vi "B_humid_air_T_2024.vi"(6 "Bdw source air-water interaction virial":i32(listbox)=3, 8 "Bw source ref water":i32(listbox)=2, 9 "Bd source ref dry air":i32(listbox)=1, 10 "xw molar fraction water vapor":dbl=0.8014618300221631 format="%.6g", 11 "Temperature (K)":dbl=373.15 format="%.4g") -> (0 "Bhumid air (xw,T) [m^3/mol]":dbl=-0.0002943870785351169, 1 "Bdw(T) [m^3/mol]":dbl=-1.3917800082878983e-05, 2 "Bw(T) [m^3/mol]":dbl=-0.00045162277028342796, 3 "Bd(T) [m^3/mol]":dbl=3.5008568678367798e-06, 4 "u(Bdw) [cm^3/mol]":dbl=1.0000812523517617 format="%_3g")   [LabVIEW 2016]
uses:
  2022/SOS_Global_2022.vi
  <vilib>/gmath/NI_Gmath.lvlib
  <vilib>/Analysis/NI_AALPro.lvlib
panel:
  out "Bdw(T) [cm^3/mol]":dbl=-13.917800082878983 format="%_6g"
  in  "interpolation method":i32(ring)=2 items=["nearest", "linear", "spline", "cubic Hermite", "Lagrange"]
  in  "interpolation method":i32(ring)=2 items=["nearest", "linear", "spline", "cubic Hermite", "Lagrange"]
  out "Bhumid air (xw,T) [cm^3/mol]":dbl=-294.38707853511687 format="%_6g"
  out "Bw(T) [cm^3/mol]":dbl=-451.62277028342794 format="%_6g"
  out "Bd(T) [cm^3/mol]":dbl=3.50085686783678
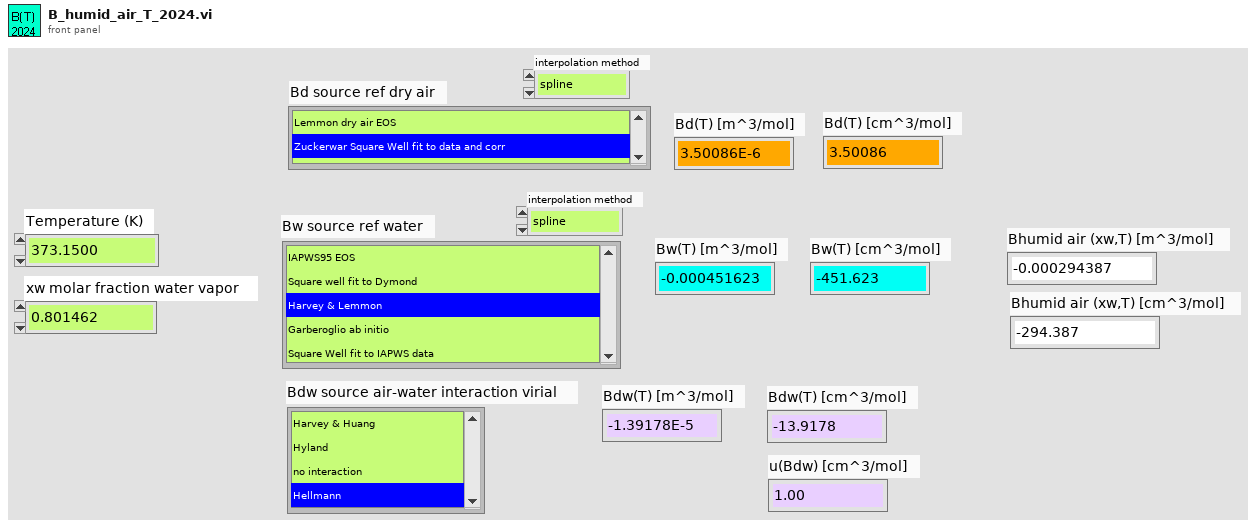
[diagram p1: front panel]
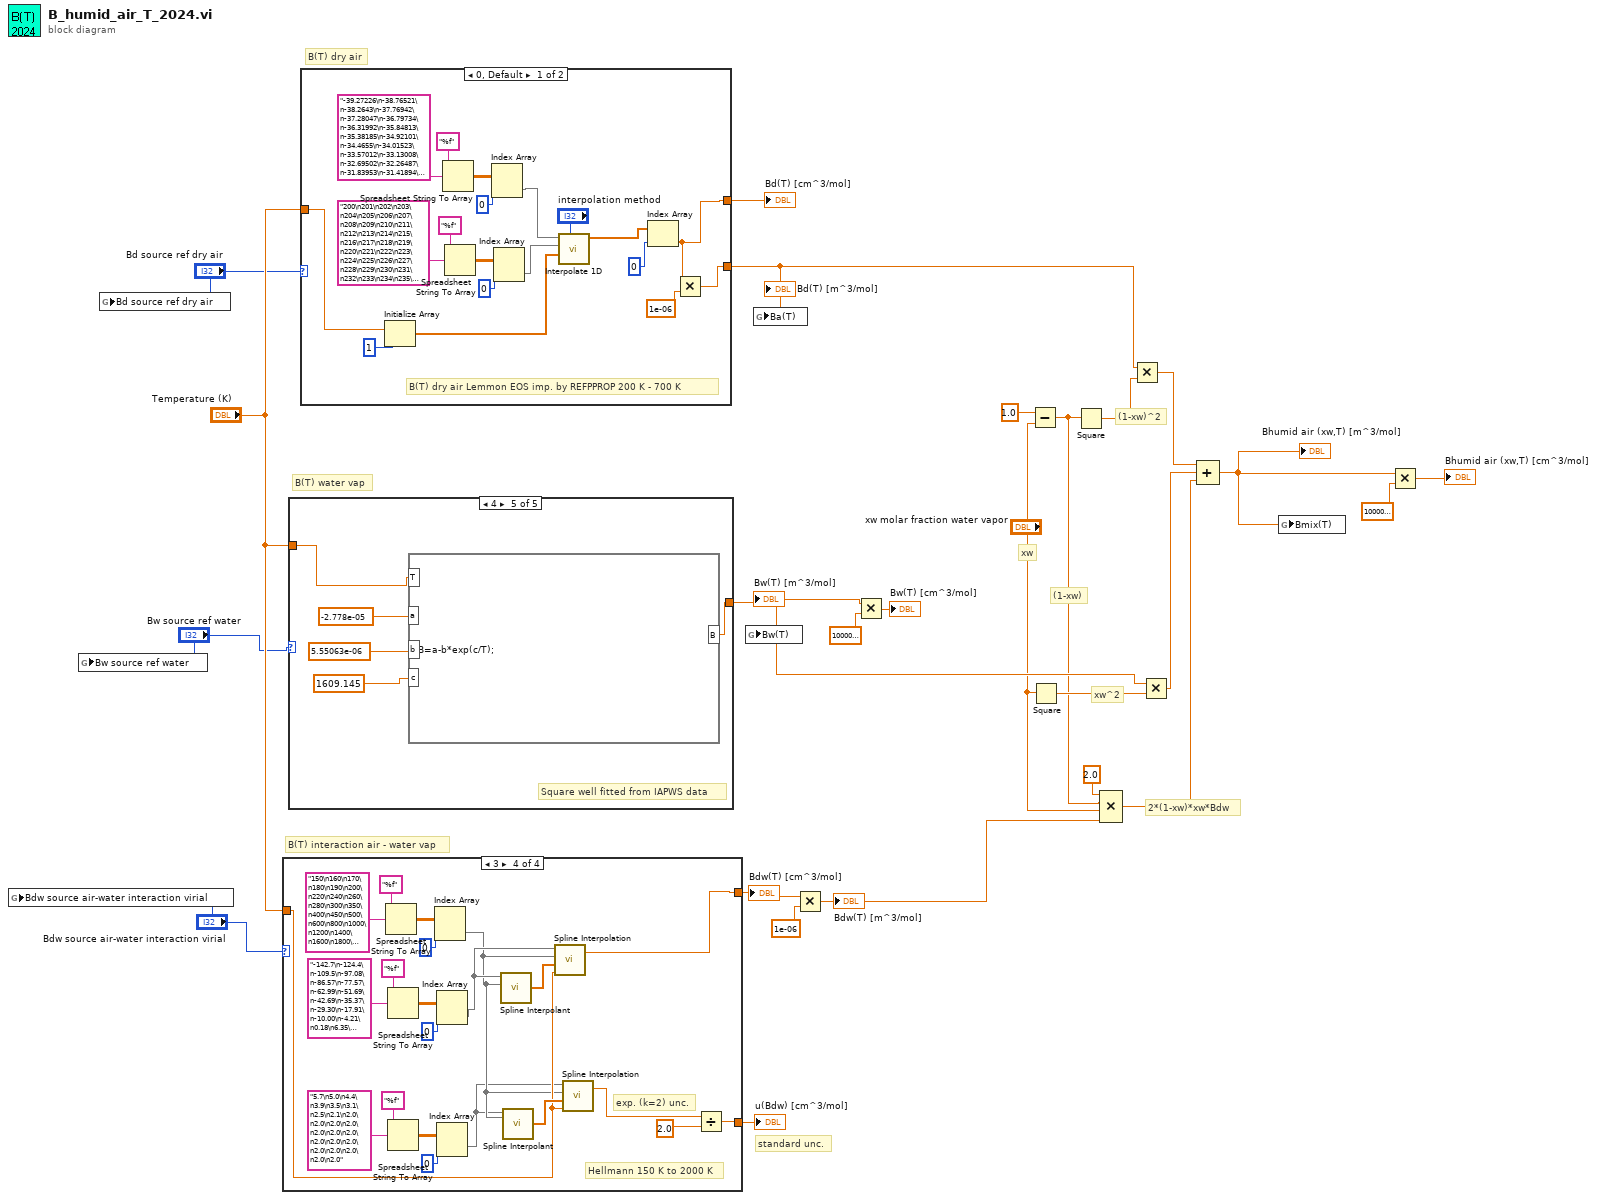
[diagram p0: block diagram]
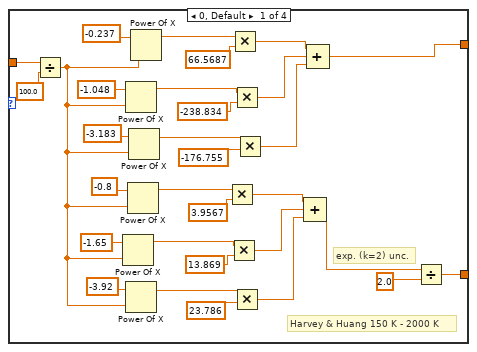
[diagram p2: hidden frame]
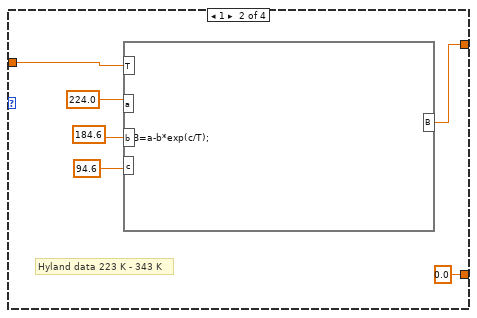
[diagram p3: hidden frame]
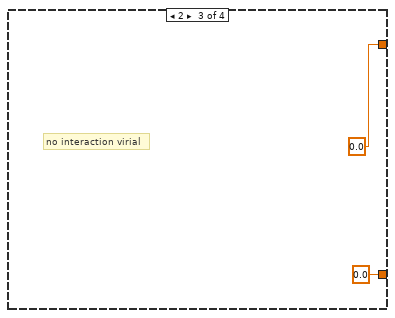
[diagram p4: hidden frame]
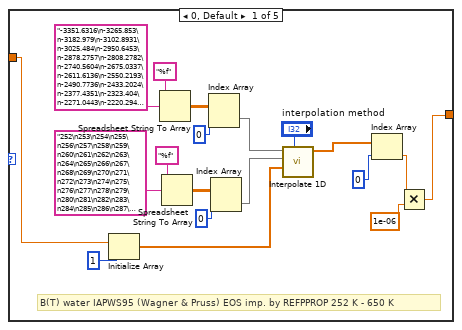
[diagram p5: hidden frame]
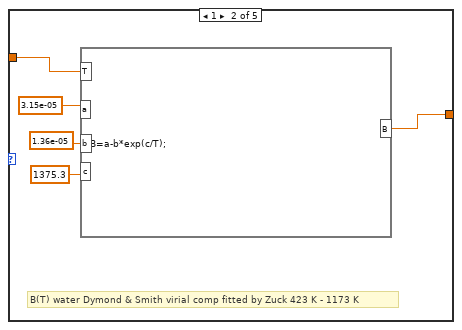
[diagram p6: hidden frame]
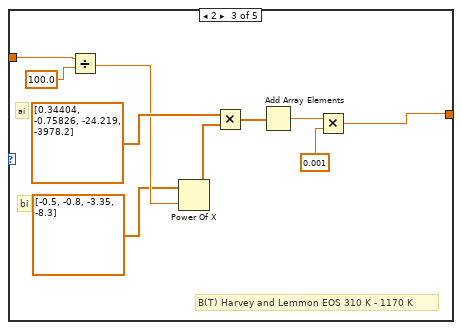
[diagram p7: hidden frame]
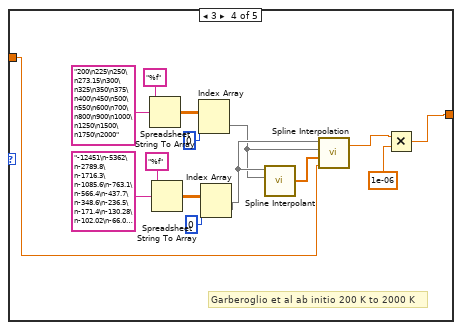
[diagram p8: hidden frame]
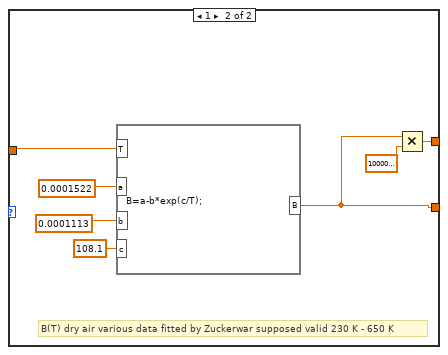
[diagram p9: hidden frame]
diagram:
  # "(1-xw)"
  # "2*(1-xw)*xw*Bdw"
  # "xw"
  # "standard unc."
  # "B(T) interaction air - water vap"
  # "xw^2"
  # "(1-xw)^2"
  # "B(T) dry air"
  # "B(T) water vap"
  n1 = global write "SOS_Global_2022.vi" "Bdw source air-water interaction virial"("Bdw source air-water interaction virial") -> ()
  n2 = global write "SOS_Global_2022.vi" "Bw source ref water"("Bw source ref water") -> ()
  n3 = global write "SOS_Global_2022.vi" "Bd source ref dry air"("Bd source ref dry air") -> ()
  n4 = case shown="3" "Bdw source air-water interaction virial" {
    tunnel: "Temperature (K)" -> [w56 w59 _ w71]
    tunnel: [w50 w58 0.0 ("B") w66] -> w7
    tunnel: [w27 0.0 0.0 w67] -> w8
    frame 0, Default {
      # "exp. (k=2) unc."
      # "Harvey & Huang 150 K - 2000 K"
      n5 = Divide(x=w56, y=100.0) -> (x/y=w29:dbl)
      n6 = Power Of X(1:w29, 2:-1.65 ("y")) -> (0:w35:dbl)
      n7 = Power Of X(1:w29, 2:-1.048 ("y")) -> (0:w47:dbl)
      n8 = Power Of X(1:w29, 2:-3.92 ("y")) -> (0:w32:dbl)
      n9 = Power Of X(1:w29, 2:-0.8 ("y")) -> (0:w40:dbl)
      n10 = Power Of X(1:w29, 2:-3.183 ("y")) -> (0:w44:dbl)
      n11 = Power Of X(1:w29, 2:-0.237 ("y")) -> (0:w53:dbl)
      n12 = Multiply(x=w40, y=3.9567) -> (x*y=w38:dbl)
      n13 = Multiply(x=w35, y=13.869) -> (x*y=w34:dbl)
      n14 = Multiply(x=w53, y=66.5687) -> (x*y=w51:dbl)
      n15 = Multiply(x=w47, y=-238.834) -> (x*y=w46:dbl)
      n16 = Multiply(x=w32, y=23.786) -> (x*y=w30:dbl)
      n17 = Multiply(x=w44, y=-176.755) -> (x*y=w42:dbl)
      n18 = Compound Arithmetic op=ADD(w38, w34, w30) -> (w28:dbl)
      n19 = Compound Arithmetic op=ADD(w51, w46, w42) -> (w50:dbl)
      n20 = Divide(x=w28, y=2.0) -> (x/y=w27:dbl)
    }
    frame 1 {
      # "Hyland data 223 K - 343 K"
      n21 = formula code="B=a-b*exp(c/T);"("T"=w59, "a"=224.0, "b"=184.6, "c"=94.6) -> ("B"=w58:dbl)
    }
    frame 2 {
      # "no interaction virial"
    }
    frame 3 {
      # "exp. (k=2) unc."
      # "Hellmann 150 K to 2000 K"
      n22 = Spreadsheet String To Array(format string="%f", spreadsheet string="150\n160\n170\n180\n190\n200\n220\n240\n260\n280\n300\n350\n400\n450\n500\n600\n800\n1000\n1200\n1400\n1600\n1800\n2000") -> (array=w78:dbl[][])  [unwired: 2 in]
      n23 = Spreadsheet String To Array(format string="%f", spreadsheet string="-142.7\n-124.4\n-109.5\n-97.08\n-86.57\n-77.57\n-62.99\n-51.69\n-42.69\n-35.37\n-29.30\n-17.91\n-10.00\n-4.21\n0.18\n6.35\n13.29\n16.93\n19.06\n20.40\n21.27\n21.84\n22.23") -> (array=w82:dbl[][])  [unwired: 2 in]
      n24 = Spreadsheet String To Array(format string="%f", spreadsheet string="5.7\n5.0\n4.4\n3.9\n3.5\n3.1\n2.5\n2.1\n2.0\n2.0\n2.0\n2.0\n2.0\n2.0\n2.0\n2.0\n2.0\n2.0\n2.0\n2.0\n2.0\n2.0\n2.0") -> (array=w74:dbl[][])  [unwired: 2 in]
      n25 = Index Array(array=w78, index (col)=0 ("disabled index (col)")) -> (element=w69:dbl[])  [unwired: 1 in]
      n26 = Index Array(array=w82, index (col)=0 ("disabled index (col)")) -> (element=w86:dbl[])  [unwired: 1 in]
      n27 = Index Array(array=w74, index (col)=0 ("disabled index (col)")) -> (element=w65:dbl[])  [unwired: 1 in]
      n28 = call <vilib>:"Spline Interpolant.vi"("X"=w69, "Y"=w86) -> ("Interpolant"=w85:dbl[])  [unwired: 2 in, 1 out]
      n29 = call <vilib>:"Spline Interpolant.vi"("X"=w69, "Y"=w65) -> ("Interpolant"=w72:dbl[])  [unwired: 2 in, 1 out]
      n30 = call <vilib>:"Spline Interpolation.vi"("x value"=w71, "Interpolant"=w85, "X"=w69, "Y"=w86) -> ("interpolation value"=w66:dbl)  [unwired: 1 out]
      n31 = call <vilib>:"Spline Interpolation.vi"("x value"=w71, "Interpolant"=w72, "X"=w69, "Y"=w65) -> ("interpolation value"=w68:dbl)  [unwired: 1 out]
      n32 = Divide(x=w68, y=2.0) -> (x/y=w67:dbl)
    }
  }
  "Bdw(T) [cm^3/mol]" <- w7
  "u(Bdw) [cm^3/mol]" <- w8
  n33 = case shown="4" "Bw source ref water" {
    tunnel: "Temperature (K)" -> [w99 w107 w120 w124 w137]
    tunnel: [w97 w106 w111 w121 w136] -> w19
    frame 0, Default {
      # "B(T) water IAPWS95 (Wagner & Pruss) EOS imp. by REFPPROP 252 K - 650 K"
      n34 = Initialize Array(w99, 1 ("dimension size")) -> (w103:dbl[])
      n35 = Spreadsheet String To Array(format string="%f", spreadsheet string="-3351.6316\n-3265.853\n-3182.979\n-3102.8931\n-3025.484\n-2950.6453\n-2878.2757\n-2808.2782\n-2740.5604\n-2675.0337\n-2611.6136\n-2550.2193\n-2490.7736\n-2433.2024\n-2377.4351\n-2323.404\n-2271.0443\n-2220.294\n-2171.0936\n-2123.3865\n-2077.1179\n-2032.2357\n-1988.6898\n-1946.4323\n-1905.4172\n-1865.6002\n-1826.9391\n-1789.3932\n-1752.9236\n-1717.4929\n-1683.065\n-1649.6055\n-1617.0813\n-1585.4606\n-1554.7126\n-1524.8081\n-1495.7188\n-1467.4174\n-1439.8779\n-1413.0752\n-1386.985\n-1361.5841\n-1336.8502\n-1312.7616\n-1289.2976\n-1266.4383\n-1244.1643\n-1222.4573\n-1201.2993\n-1180.6731\n-1160.5622\n-1140.9505\n-1121.8228\n-1103.164\n-1084.96\n-1067.1968\n-1049.8612\n-1032.9402\n-1016.4216\n-1000.2932\n-984.54359\n-969.16154\n-954.13627\n-939.45738\n-925.1148\n-911.09882\n-897.40004\n-884.0094\n-870.91812\n-858.11771\n-845.59999\n-833.35702\n-821.38114\n-809.66492\n-798.2012\n-786.98303\n-776.0037\n-765.25669\n-754.73573\n-744.43471\n-734.34773\n-724.46907\n-714.79322\n-705.3148\n-696.02862\n-686.92965\n-678.01302\n-669.27399\n-660.70798\n-652.31057\n-644.07743\n-636.00439\n-628.08741\n-620.32255\n-612.706\n-605.23407\n-597.90317\n-590.70981\n-583.65063\n-576.72233\n-569.92173\n-563.24575\n-556.69137\n-550.25568\n-543.93585\n-537.72913\n-531.63285\n-525.6444\n-519.76126\n-513.98098\n-508.30118\n-502.71953\n-497.23378\n-491.84174\n-486.54128\n-481.33032\n-476.20686\n-471.16892\n-466.2146\n-461.34205\n-456.54945\n-451.83504\n-447.19713\n-442.63403\n-438.14413\n-433.72584\n-429.37763\n-425.09801\n-420.8855\n-416.7387\n-412.65621\n-408.63669\n-404.67882\n-400.78132\n-396.94294\n-393.16247\n-389.43872\n-385.77053\n-382.15678\n-378.59636\n-375.08821\n-371.63127\n-368.22453\n-364.86699\n-361.55769\n-358.29567\n-355.08\n-351.9098\n-348.78417\n-345.70225\n-342.66322\n-339.66625\n-336.71053\n-333.7953\n-330.91978\n-328.08323\n-325.28492\n-322.52415\n-319.80022\n-317.11245\n-314.46018\n-311.84275\n-309.25955\n-306.70994\n-304.19333\n-301.70912\n-299.25674\n-296.83561\n-294.4452\n-292.08495\n-289.75434\n-287.45285\n-285.17998\n-282.93524\n-280.71813\n-278.52818\n-276.36494\n-274.22795\n-272.11676\n-270.03094\n-267.97007\n-265.93373\n-263.92151\n-261.93301\n-259.96785\n-258.02564\n-256.106\n-254.20858\n-252.333\n-250.47892\n-248.646\n-246.8339\n-245.04228\n-243.27082\n-241.5192\n-239.78712\n-238.07426\n-236.38033\n-234.70504\n-233.04809\n-231.40921\n-229.78812\n-228.18454\n-226.59822\n-225.02889\n-223.4763\n-221.94019\n-220.42032\n-218.91645\n-217.42834\n-215.95576\n-214.49849\n-213.05629\n-211.62895\n-210.21626\n-208.81799\n-207.43396\n-206.06394\n-204.70775\n-203.36518\n-202.03604\n-200.72015\n-199.41732\n-198.12736\n-196.8501\n-195.58536\n-194.33297\n-193.09275\n-191.86455\n-190.64819\n-189.44352\n-188.25038\n-187.06861\n-185.89806\n-184.73858\n-183.59003\n-182.45225\n-181.3251\n-180.20846\n-179.10217\n-178.0061\n-176.92012\n-175.8441\n-174.77791\n-173.72142\n-172.67451\n-171.63706\n-170.60894\n-169.59004\n-168.58024\n-167.57943\n-166.58749\n-165.60432\n-164.6298\n-163.66382\n-162.70629\n-161.75709\n-160.81613\n-159.88331\n-158.95852\n-158.04167\n-157.13265\n-156.23139\n-155.33778\n-154.45174\n-153.57316\n-152.70198\n-151.83808\n-150.9814\n-150.13185\n-149.28933\n-148.45378\n-147.62511\n-146.80324\n-145.98809\n-145.17958\n-144.37764\n-143.58219\n-142.79316\n-142.01048\n-141.23407\n-140.46386\n-139.69979\n-138.94179\n-138.18978\n-137.4437\n-136.70348\n-135.96907\n-135.24039\n-134.51739\n-133.79999\n-133.08815\n-132.3818\n-131.68087\n-130.98532\n-130.29508\n-129.6101\n-128.93032\n-128.25568\n-127.58614\n-126.92163\n-126.2621\n-125.6075\n-124.95779\n-124.3129\n-123.67279\n-123.03741\n-122.4067\n-121.78063\n-121.15914\n-120.54219\n-119.92972\n-119.3217\n-118.71808\n-118.11881\n-117.52386\n-116.93317\n-116.3467\n-115.76441\n-115.18627\n-114.61222\n-114.04223\n-113.47625\n-112.91426\n-112.3562\n-111.80204\n-111.25175\n-110.70528\n-110.16259\n-109.62366\n-109.08844\n-108.5569\n-108.029\n-107.50471\n-106.98399\n-106.46682\n-105.95314\n-105.44294\n-104.93618\n-104.43283\n-103.93285\n-103.43622\n-102.9429\n-102.45286\n-101.96607\n-101.4825\n-101.00212\n-100.5249\n-100.05082\n-99.57984\n-99.11194\n-98.64708\n-98.18524\n-97.72639\n-97.27052\n-96.81757\n-96.36755\n-95.9204\n-95.47612\n-95.03467\n-94.59603\n-94.16017\n-93.72708\n-93.29672\n-92.86907\n-92.44411\n-92.02181\n-91.60216\n-91.18512\n-90.77067\n-90.3588\n-89.94948\n-89.54269\n-89.1384\n-88.73659\n-88.33726\n-87.94036\n-87.54588\n-87.15381\n-86.76412\n-86.37678\n-85.99179\n-85.60912\n-85.22875\n-84.85067\n-84.47484\n-84.10126\n-83.72991\n-83.36076\n-82.9938\n-82.62901\n-82.26638\n-81.90588\n-81.5475\n-81.19122\n-80.83702\n-80.48489\n-80.13481\n-79.78676") -> (array=w92:dbl[][])  [unwired: 2 in]
      n36 = Spreadsheet String To Array(format string="%f", spreadsheet string="252\n253\n254\n255\n256\n257\n258\n259\n260\n261\n262\n263\n264\n265\n266\n267\n268\n269\n270\n271\n272\n273\n274\n275\n276\n277\n278\n279\n280\n281\n282\n283\n284\n285\n286\n287\n288\n289\n290\n291\n292\n293\n294\n295\n296\n297\n298\n299\n300\n301\n302\n303\n304\n305\n306\n307\n308\n309\n310\n311\n312\n313\n314\n315\n316\n317\n318\n319\n320\n321\n322\n323\n324\n325\n326\n327\n328\n329\n330\n331\n332\n333\n334\n335\n336\n337\n338\n339\n340\n341\n342\n343\n344\n345\n346\n347\n348\n349\n350\n351\n352\n353\n354\n355\n356\n357\n358\n359\n360\n361\n362\n363\n364\n365\n366\n367\n368\n369\n370\n371\n372\n373\n374\n375\n376\n377\n378\n379\n380\n381\n382\n383\n384\n385\n386\n387\n388\n389\n390\n391\n392\n393\n394\n395\n396\n397\n398\n399\n400\n401\n...") -> (array=w95:dbl[][])  [unwired: 2 in]
      n37 = Index Array(array=w92, index (col)=0 ("disabled index (col)")) -> (element=w87:dbl[])  [unwired: 1 in]
      n38 = Index Array(array=w95, index (col)=0 ("disabled index (col)")) -> (element=w88:dbl[])  [unwired: 1 in]
      n39 = call <vilib>:"Interpolate 1D.vi"("method"="interpolation method", "xi"=w103, "X"=w88, "Y"=w87) -> ("yi"=w101:dbl[])  [unwired: 5 in, 2 out]
      n40 = Index Array(array=w101, index=0) -> (element=w98:dbl)
      n41 = Multiply(x=w98, y=1e-06) -> (x*y=w97:dbl)
    }
    frame 1 {
      # "B(T) water Dymond & Smith virial comp fitted by Zuck 423 K - 1173 K"
      n42 = formula code="B=a-b*exp(c/T);"("T"=w107, "a"=3.15e-05, "b"=1.36e-05, "c"=1375.3) -> ("B"=w106:dbl)
    }
    frame 2 {
      # "bi"
      # "ai"
      # "B(T) Harvey and Lemmon EOS 310 K - 1170 K"
      n43 = Divide(x=w120, y=100.0) -> (x/y=w117:dbl)
      n44 = Power Of X(1:w117, 2:dbl[] [-0.5, -0.8, -3.35, -8.3]) -> (0:w115:dbl[])
      n45 = Multiply(x=dbl[] [0.34404, -0.75826, -24.219, -3978.2], y=w115) -> (x*y=w114:dbl[])
      n46 = Add Array Elements(numeric array=w114) -> (sum=w112:dbl)
      n47 = Multiply(x=w112, y=0.001) -> (x*y=w111:dbl)
    }
    frame 3 {
      # "Garberoglio et al ab initio 200 K to 2000 K"
      n48 = Spreadsheet String To Array(format string="%f", spreadsheet string="200\n225\n250\n273.15\n300\n325\n350\n375\n400\n450\n500\n550\n600\n700\n800\n900\n1000\n1250\n1500\n1750\n2000") -> (array=w126:dbl[][])  [unwired: 2 in]
      n49 = Spreadsheet String To Array(format string="%f", spreadsheet string="-12451\n-5362\n-2789.8\n-1716.3\n-1085.6\n-763.1\n-566.4\n-437.7\n-348.6\n-236.5\n-171.4\n-130.28\n-102.02\n-66.05\n-44.6\n-31.74\n-22.4\n-8.66\n-1.00\n3.8\n5.79") -> (array=w130:dbl[][])  [unwired: 2 in]
      n50 = Index Array(array=w126, index (col)=0 ("disabled index (col)")) -> (element=w133:dbl[])  [unwired: 1 in]
      n51 = Index Array(array=w130, index (col)=0 ("disabled index (col)")) -> (element=w135:dbl[])  [unwired: 1 in]
      n52 = call <vilib>:"Spline Interpolant.vi"("X"=w133, "Y"=w135) -> ("Interpolant"=w134:dbl[])  [unwired: 2 in, 1 out]
      n53 = call <vilib>:"Spline Interpolation.vi"("x value"=w124, "Interpolant"=w134, "X"=w133, "Y"=w135) -> ("interpolation value"=w122:dbl)  [unwired: 1 out]
      n54 = Multiply(x=w122, y=1e-06) -> (x*y=w121:dbl)
    }
    frame 4 {
      # "Square well fitted from IAPWS data"
      n55 = formula code="B=a-b*exp(c/T);"("T"=w137, "a"=-2.778e-05, "b"=5.55063e-06, "c"=1609.145) -> ("B"=w136:dbl)
    }
  }
  "Bw(T) [m^3/mol]" <- w19
  n56 = case shown="0, Default" "Bd source ref dry air" {
    tunnel: "Temperature (K)" -> [w158 w163]
    tunnel: [w154 w160] -> w13
    tunnel: [w151 w161] -> w14
    frame 0, Default {
      # "B(T) dry air Lemmon EOS imp. by REFPPROP 200 K - 700 K"
      n57 = Initialize Array(w158, 1 ("dimension size")) -> (w156:dbl[])
      n58 = Spreadsheet String To Array(format string="%f", spreadsheet string="-39.27226\n-38.76521\n-38.2643\n-37.76942\n-37.28047\n-36.79734\n-36.31992\n-35.84813\n-35.38185\n-34.92101\n-34.4655\n-34.01523\n-33.57012\n-33.13008\n-32.69502\n-32.26487\n-31.83953\n-31.41894\n-31.00301\n-30.59167\n-30.18485\n-29.78246\n-29.38445\n-28.99075\n-28.60127\n-28.21597\n-27.83476\n-27.4576\n-27.08441\n-26.71514\n-26.34972\n-25.9881\n-25.63022\n-25.27602\n-24.92545\n-24.57846\n-24.23498\n-23.89498\n-23.55839\n-23.22517\n-22.89527\n-22.56864\n-22.24523\n-21.925\n-21.60791\n-21.2939\n-20.98294\n-20.67498\n-20.36998\n-20.0679\n-19.76869\n-19.47233\n-19.17876\n-18.88795\n-18.59987\n-18.31448\n-18.03173\n-17.7516\n-17.47405\n-17.19905\n-16.92655\n-16.65654\n-16.38897\n-16.12382\n-15.86105\n-15.60063\n-15.34254\n-15.08673\n-14.83319\n-14.58188\n-14.33278\n-14.08585\n-13.84108\n-13.59843\n-13.35787\n-13.11939\n-12.88295\n-12.64853\n-12.41611\n-12.18566\n-11.95715\n-11.73057\n-11.50588\n-11.28308\n-11.06213\n-10.84301\n-10.6257\n-10.41018\n-10.19643\n-9.984431\n-9.774155\n-9.565587\n-9.358706\n-9.153492\n-8.949926\n-8.74799\n-8.547665\n-8.348932\n-8.151774\n-7.956172\n-7.76211\n-7.569569\n-7.378533\n-7.188985\n-7.000908\n-6.814287\n-6.629105\n-6.445346\n-6.262995\n-6.082036\n-5.902455\n-5.724236\n-5.547365\n-5.371827\n-5.197607\n-5.024693\n-4.85307\n-4.682724\n-4.513641\n-4.34581\n-4.179215\n-4.013845\n-3.849686\n-3.686727\n-3.524954\n-3.364355\n-3.204919\n-3.046633\n-2.889486\n-2.733466\n-2.578561\n-2.424761\n-2.272054\n-2.120429\n-1.969875\n-1.820382\n-1.671939\n-1.524536\n-1.378162\n-1.232807\n-1.088461\n-0.9451149\n-0.8027581\n-0.6613813\n-0.5209748\n-0.3815294\n-0.2430356\n-0.1054845\n0.03113316\n0.1668262\n0.3016034\n0.4354735\n0.5684451\n0.7005267\n0.8317267\n0.9620533\n1.091515\n1.220119\n1.347874\n1.474788\n1.600869\n1.726123\n1.85056\n1.974185\n2.097008\n2.219034\n2.340272\n2.460728\n2.58041\n2.699324\n2.817478\n2.934877\n3.05153\n3.167442\n3.282621\n3.397072\n3.510802\n3.623817\n3.736124\n3.84773\n3.958639\n4.068858\n4.178394\n4.287251\n4.395436\n4.502955\n4.609814\n4.716018\n4.821572\n4.926482\n5.030754\n5.134394\n5.237406\n5.339795\n5.441568\n5.542728\n5.643282\n5.743235\n5.84259\n5.941354\n6.039532\n6.137127\n6.234145\n6.330591\n6.426469\n6.521785\n6.616541\n6.710744\n6.804397\n6.897506\n6.990074\n7.082105\n7.173605\n7.264577\n7.355026\n7.444955\n7.53437\n7.623273\n7.71167\n7.799563\n7.886957\n7.973857\n8.060265\n8.146186\n8.231623\n8.31658\n8.401062\n8.48507\n8.568611\n8.651686\n8.734299\n8.816455\n8.898156\n8.979406\n9.060209\n9.140567\n9.220484\n9.299964\n9.37901\n9.457625\n9.535812\n9.613575\n9.690917\n9.76784\n9.844348\n9.920445\n9.996132\n10.07141\n10.14629\n10.22077\n10.29485\n10.36854\n10.44184\n10.51475\n10.58727\n10.65941\n10.73117\n10.80255\n10.87356\n10.9442\n11.01446\n11.08437\n11.1539\n11.22308\n11.2919\n11.36036\n11.42847\n11.49622\n11.56363\n11.63069\n11.69741\n11.76379\n11.82983\n11.89553\n11.96089\n12.02593\n12.09063\n12.15501\n12.21907\n12.2828\n12.34621\n12.4093\n12.47207\n12.53454\n12.59669\n12.65853\n12.72006\n12.78128\n12.84221\n12.90283\n12.96315\n13.02318\n13.08291\n13.14234\n13.20149\n13.26034\n13.31891\n13.37719\n13.43519\n13.4929\n13.55034\n13.6075\n13.66438\n13.72099\n13.77732\n13.83338\n13.88918\n13.94471\n13.99997\n14.05496\n14.1097\n14.16417\n14.21839\n14.27235\n14.32605\n14.3795\n14.43269\n14.48564\n14.53834\n14.59078\n14.64299\n14.69495\n14.74666\n14.79814\n14.84937\n14.90037\n14.95113\n15.00165\n15.05194\n15.102\n15.15183\n15.20143\n15.2508\n15.29994\n15.34886\n15.39756\n15.44603\n15.49428\n15.54231\n15.59012\n15.63772\n15.6851\n15.73227\n15.77922\n15.82596\n15.87249\n15.91881\n15.96493\n16.01083\n16.05654\n16.10203\n16.14733\n16.19242\n16.23731\n16.282\n16.3265\n16.3708\n16.4149\n16.4588\n16.50252\n16.54604\n16.58937\n16.63251\n16.67546\n16.71822\n16.7608\n16.80319\n16.8454\n16.88742\n16.92926\n16.97092\n17.01239\n17.05369\n17.09481\n17.13576\n17.17652\n17.21712\n17.25753\n17.29778\n17.33785\n17.37775\n17.41748\n17.45704\n17.49644\n17.53566\n17.57472\n17.61362\n17.65235\n17.69091\n17.72932\n17.76756\n17.80564\n17.84356\n17.88132\n17.91892\n17.95637\n17.99366\n18.03079\n18.06777\n18.1046\n18.14127\n18.17779\n18.21416\n18.25038\n18.28645\n18.32237\n18.35814\n18.39377\n18.42925\n18.46458\n18.49977\n18.53481\n18.56971\n18.60447\n18.63909\n18.67357\n18.7079\n18.7421\n18.77615\n18.81007\n18.84386\n18.8775\n18.91101\n18.94439\n18.97763\n19.01074\n19.04371\n19.07656\n19.10927\n19.14185\n19.1743\n19.20662\n19.23881\n19.27087\n19.30281\n19.33462\n19.36631\n19.39786\n19.4293\n19.46061\n19.4918\n19.52286\n19.5538\n19.58462\n19.61532\n19.6459\n19.67636\n19.7067\n19.73692\n19.76702\n19.79701\n19.82688\n19.85664\n19.88627\n19.9158\n19.94521\n19.9745\n20.00369\n20.03276\n20.06172\n20.09056\n20.1193\n20.14792\n20.17644\n20.20485\n20.23315\n20.26134\n20.28942\n20.3174\n20.34526\n20.37303\n20.40069\n20.42824\n20.45569\n20.48303\n20.51027\n20.53741\n20.56445\n20.59138\n20.61822\n20.64495\n20.67158\n20.69811\n20.72455\n20.75088\n20.77712\n20.80325\n20.82929\n20.85524\n20.88108\n20.90684\n20.93249\n20.95805\n20.98352\n21.00889\n21.03416\n21.05935\n21.08444\n21.10944\n21.13435\n21.15916") -> (array=w146:dbl[][])  [unwired: 2 in]
      n59 = Spreadsheet String To Array(format string="%f", spreadsheet string="200\n201\n202\n203\n204\n205\n206\n207\n208\n209\n210\n211\n212\n213\n214\n215\n216\n217\n218\n219\n220\n221\n222\n223\n224\n225\n226\n227\n228\n229\n230\n231\n232\n233\n234\n235\n236\n237\n238\n239\n240\n241\n242\n243\n244\n245\n246\n247\n248\n249\n250\n251\n252\n253\n254\n255\n256\n257\n258\n259\n260\n261\n262\n263\n264\n265\n266\n267\n268\n269\n270\n271\n272\n273\n274\n275\n276\n277\n278\n279\n280\n281\n282\n283\n284\n285\n286\n287\n288\n289\n290\n291\n292\n293\n294\n295\n296\n297\n298\n299\n300\n301\n302\n303\n304\n305\n306\n307\n308\n309\n310\n311\n312\n313\n314\n315\n316\n317\n318\n319\n320\n321\n322\n323\n324\n325\n326\n327\n328\n329\n330\n331\n332\n333\n334\n335\n336\n337\n338\n339\n340\n341\n342\n343\n344\n345\n346\n347\n348\n349\n...") -> (array=w149:dbl[][])  [unwired: 2 in]
      n60 = Index Array(array=w146, index (col)=0 ("disabled index (col)")) -> (element=w141:dbl[])  [unwired: 1 in]
      n61 = Index Array(array=w149, index (col)=0 ("disabled index (col)")) -> (element=w142:dbl[])  [unwired: 1 in]
      n62 = call <vilib>:"Interpolate 1D.vi"("method"="interpolation method", "xi"=w156, "X"=w142, "Y"=w141) -> ("yi"=w153:dbl[])  [unwired: 5 in, 2 out]
      n63 = Index Array(array=w153, index=0) -> (element=w151:dbl)
      n64 = Multiply(x=w151, y=1e-06) -> (x*y=w154:dbl)
    }
    frame 1 {
      # "B(T) dry air various data fitted by Zuckerwar supposed valid 230 K - 650 K"
      n65 = formula code="B=a-b*exp(c/T);"("T"=w163, "a"=0.0001522, "b"=0.0001113, "c"=108.1) -> ("B"=w160:dbl)
      n66 = Multiply(x=w160, y=1000000.0) -> (x*y=w161:dbl)
    }
  }
  "Bd(T) [m^3/mol]" <- w13
  "Bd(T) [cm^3/mol]" <- w14
  n67 = global write "SOS_Global_2022.vi" "Bw(T)"(w19) -> ()
  n68 = global write "SOS_Global_2022.vi" "Ba(T)"(w13) -> ()
  n69 = Multiply(x=w7, y=1e-06) -> (x*y=w4:dbl)
  "Bdw(T) [m^3/mol]" <- w4
  n70 = Multiply(x=w19, y=1000000.0) -> (x*y=→"Bw(T) [cm^3/mol]":dbl)
  n71 = Subtract(x=1.0, y="xw molar fraction water vapor") -> (x-y=w6:dbl)
  n72 = Square(x="xw molar fraction water vapor") -> (x^2=w23:dbl)
  n73 = Square(x=w6) -> (x^2=w24:dbl)
  n74 = Compound Arithmetic op=MULTIPLY(2.0 ("value"), w6, "xw molar fraction water vapor", w4) -> (w9:dbl)
  n75 = Multiply(x=w13, y=w24) -> (x*y=w22:dbl)
  n76 = Multiply(x=w19, y=w23) -> (x*y=w21:dbl)
  n77 = Compound Arithmetic op=ADD(w22, w21, w9) -> (w16:dbl)
  "Bhumid air (xw,T) [m^3/mol]" <- w16
  n78 = global write "SOS_Global_2022.vi" "Bmix(T)"(w16) -> ()
  n79 = Multiply(x=w16, y=1000000.0) -> (x*y=→"Bhumid air (xw,T) [cm^3/mol]":dbl)
